vi "Array_Investigation Part 2.vi"() -> ()   [LabVIEW 2014]
doc: "This VI is an exercise in the LabVIEW Core I course.\n\nEnter the number of columns and rows you want generated, then run the VI. This VI generates an array with the number of rows and columns you specify."
panel:
  out "Intensity Graph":dbl[][](graph)
  out "Array":dbl[][](array[numeric])
  in  "Rows":i32=80
  in  "Columns":i32=80
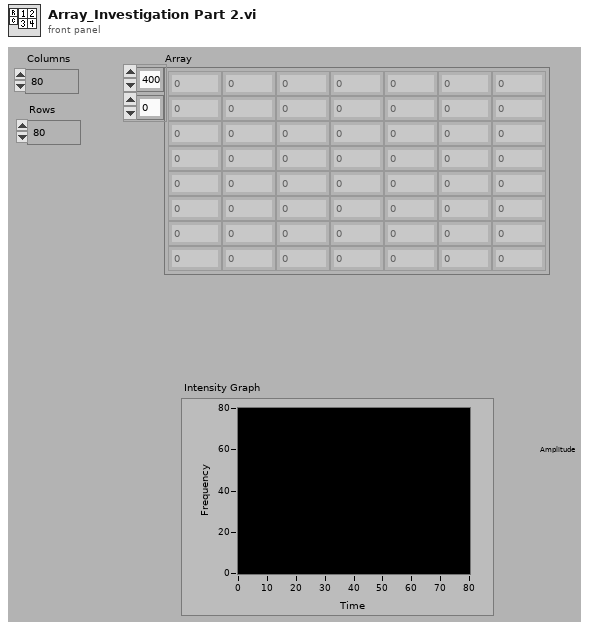
[diagram p1: front panel]
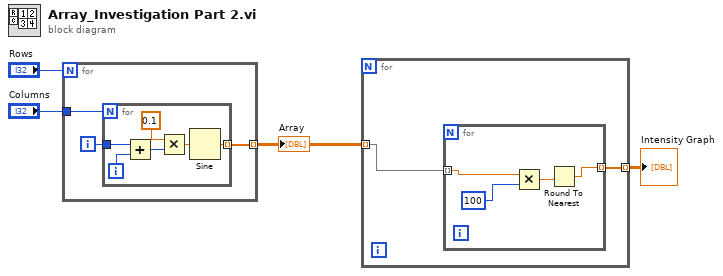
[diagram p0: block diagram]
diagram:
  n1 = for {
    N: "Rows" -> [_]
    tunnel: [w7] -> w2 mode=indexing
    tunnel: "Columns" -> [w6]
    i -> [w5]
    n2 = for {
      N: w6 -> [_]
      tunnel: [w13] -> w7 mode=indexing
      tunnel: w5 -> [w10]
      i -> [w11]
      n3 = Add(x=w10, y=w11) -> (x+y=w12:i32)
      n4 = Multiply(x=0.1, y=w12) -> (x*y=w9:dbl)
      n5 = Sine(x=w9) -> (sin(x)=w13:dbl)
    }
  }
  "Array" <- w2
  n6 = for {
    tunnel: w2 -> [w15] mode=indexing
    tunnel: [w14] -> w1 mode=indexing
    n7 = for {
      tunnel: w15 -> [w18] mode=indexing
      tunnel: [w16] -> w14 mode=indexing
      n8 = Multiply(x=w18, y=100) -> (x*y=w17:dbl)
      n9 = Round To Nearest(number=w17) -> (nearest integer value=w16:dbl)
    }
  }
  "Intensity Graph" <- w1
